vi "inferenz4.vi"(0 "fuzzified input 1":T1={"index"=-1, "fulfillment"=[], "active sets"=[3]} {"fulfillment" min=0.0 max=1.0 step=0.01 format="%.2f"}, 1 "fuzzified input 2":T1={"index"=-1, "fulfillment"=[], "active sets"=[3]} {"fulfillment" min=0.0 max=1.0 step=0.01 format="%.2f"}, 2 "fuzzified input 3":T1={"index"=-1, "fulfillment"=[], "active sets"=[3]} {"fulfillment" min=0.0 max=1.0 step=0.01 format="%.2f"}, 3 "fuzzified input 4":T1={"index"=-1, "fulfillment"=[], "active sets"=[3]} {"fulfillment" min=0.0 max=1.0 step=0.01 format="%.2f"}, 4 "Controller":T3={"Parameters"={"antecedance"=[{"ling.var."="in1", "x-min"=-1.0, "x-max"=1.0, "setarray"=[{"linguistic term"="NE1", "color"=16711680, "points"=[-1.0, -1.0, -1.0, -2.2351741790771484e-05]}, {"linguistic term"="ZE1", "color"=255, "points"=[-1.0, 0.0, 0.0, 1.0]}, {"linguistic term"="PO1", "color"=26214, "points"=[0.0, 1.0, 1.0, 1.0]}, {"linguistic term"="PB1", "color"=0, "points"=[0.009999999776482582, 0.009999999776482582, 0.009999999776482582, 0.009999999776482582]}]}, {"ling.var."="in2", "x-min"=-1.0, "x-max"=1.0, "setarray"=[{"linguistic term"="NE2", "color"=0, "points"=[0.0, 0.009999999776482582, 0.009999999776482582, 0.009999999776482582]}, {"linguistic term"="PO2", "color"=0, "points"=[0.0, 0.009999999776482582, 0.009999999776482582, 0.009999999776482582]}]}, {"ling.var."="in3", "x-min"=-1.0, "x-max"=1.0, "setarray"=[{"linguistic term"="NE1", "color"=0, "points"=[-1.0, -1.0000001192092896, -1.0000001192092896, 0.0]}, {"linguistic term"="ZE1", "color"=0, "points"=[-1.0000001192092896, 0.0, 0.0, 1.0000001192092896]}, {"linguistic term"="PO1", "color"=0, "points"=[1.4901161193847656e-08, 1.0, 1.0, 1.0000001192092896]}]}], "consequence"=[{"ling.var."="out", "x-min"=-1.0, "x-max"=1.0, "setarray"=[{"linguistic term"="NEo", "color"=16711680, "points"=[-1.0, -1.0, -1.0, 0.0]}, {"linguistic term"="ZEo", "color"=255, "points"=[-1.0, 0.0, 0.0, 1.0]}, {"linguistic term"="POo", "color"=26214, "points"=[0.0, 1.0, 1.0, 1.0]}]}], "conclusions"=[0, 1, 2, 0, 1, 2, 0, 1, 2, 2, 2, 2, 0, 0, 0, 1, 1, 1, 2, 1, 0, 2, 1, 0], "degree-of-support"=[1.0, 1.0, 1.0, 1.0, 1.0, 1.0, 1.0], "defu"=[{"inference"=0, "defumethod"=0, "modification"=TRUE, "precision"=0, "no consequence"=0, "defaultvalue"=0.0}]}, "Description"={"Info"={"Path"=path "/HD 1000/Desktop Folder/fuzzylab today/loadsave.vi", "Controller Name"="", "Date"="", "Time"=""}, "Author"="", "Text"=""}} {"Parameters"."defu"."defaultvalue" format="%.2f"; "Parameters"."degree-of-support" step=0.009999999776482582 format="%.2f"; "Parameters"."consequence"."x-min" step=0.009999999776482582 format="%.2f"; "Parameters"."consequence"."x-max" step=0.009999999776482582 format="%.2f"; "Parameters"."consequence"."setarray"."points" step=0.009999999776482582 format="%.2f"; "Parameters"."antecedance"."x-min" step=0.009999999776482582 format="%.2f"; "Parameters"."antecedance"."x-max" step=0.009999999776482582 format="%.2f"; "Parameters"."antecedance"."setarray"."points" step=0.009999999776482582 format="%.2f"}) -> (5 "fuzzified consequence":T2={"fullfilment*DoS"=[19.0, 20.0, 22.0, 23.0], "active consequence"=[19, 20, 22, 23]} {"fullfilment*DoS" format="%.2f"}, 6 "firering rules":i32[](array[numeric])=[19, 20, 22, 23], 7 "error out":errorcluster={"status"=FALSE, "code"=0, "source"="no error"})   [LabVIEW 2020, in "NI_fuzzy logic.lvlib"]
uses:
  <vilib>/addons/control/fuzzy/NI_fuzzy logic.lvlib
panel:
  in  "no error":errorcluster
  out "Minimum":dbl[](array[numeric])=[19.0, 20.0, 22.0, 23.0] format="%.2f"
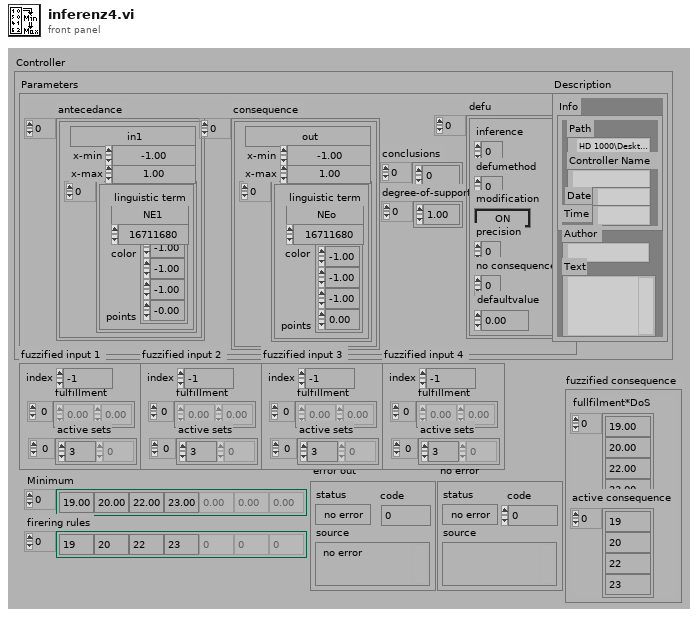
[diagram p1: front panel]
types:
  T1 = cluster{"index":i32, "fulfillment":dbl[], "active sets":i32[]}
  T2 = cluster{"fullfilment*DoS":dbl[], "active consequence":i32[]}
  T3 = cluster{"Parameters":cluster{"antecedance":cluster{"ling.var.":string, "x-min":dbl, "x-max":dbl, "setarray":cluster{"linguistic term":string, "color":u32, "points":dbl[]}[]}[], "consequence":cluster{"ling.var.":string, "x-min":dbl, "x-max":dbl, "setarray":cluster{"linguistic term":string, "color":u32, "points":dbl[]}[]}[], "conclusions":u16[], "degree-of-support":dbl[], "defu":cluster{"inference":u16, "defumethod":u16, "modification":bool, "precision":u16, "no consequence":u16, "defaultvalue":dbl}[]}, "Description":cluster{"Info":cluster{"Path":path, "Controller Name":string, "Date":string, "Time":string}, "Author":string, "Text":string}}
  T4 = cluster{"index":i32, "fulfillment":dbl[], "active sets":i32[]}[]
  T5 = cluster{"ling.var.":string, "x-min":dbl, "x-max":dbl, "setarray":cluster{"linguistic term":string, "color":u32, "points":dbl[]}[]}[]
  T6 = cluster{"ling.var.":string, "x-min":dbl, "x-max":dbl, "setarray":cluster{"linguistic term":string, "color":u32, "points":dbl[]}[]}
  T7 = cluster{"linguistic term":string, "color":u32, "points":dbl[]}[]
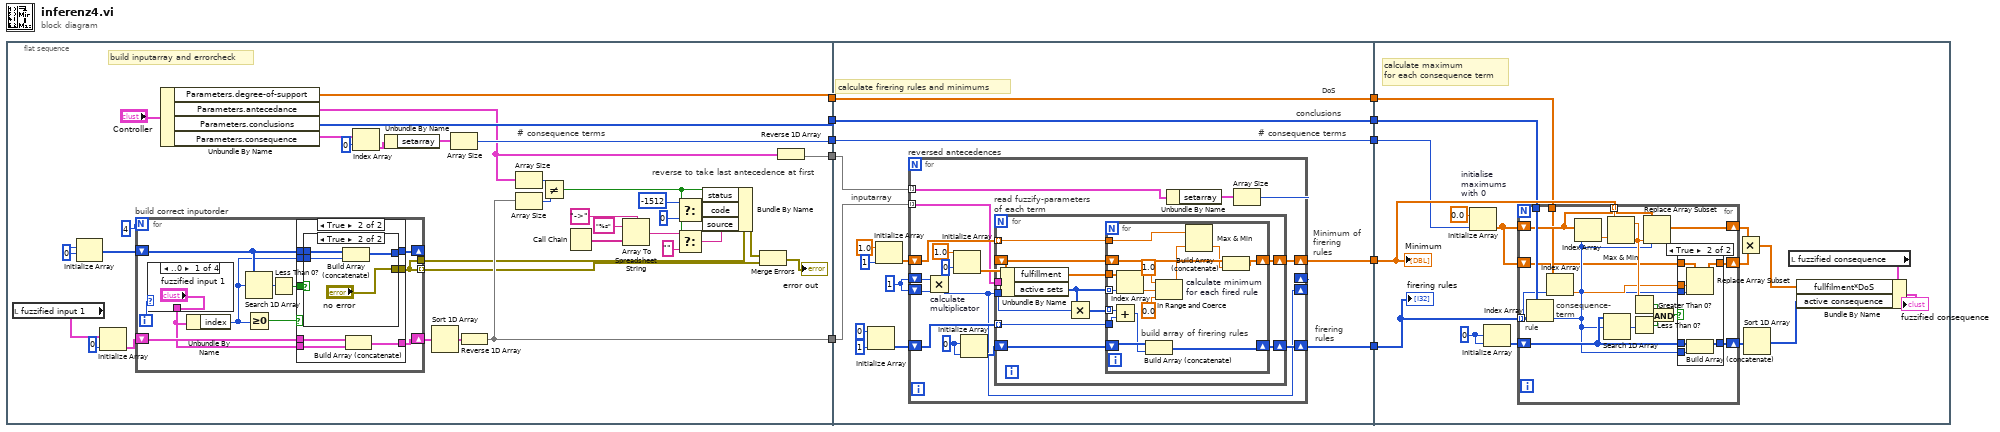
[diagram p0: block diagram]
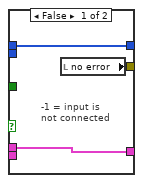
[diagram p2: hidden frame]
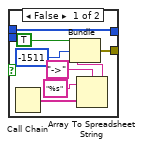
[diagram p3: hidden frame]
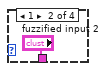
[diagram p4: hidden frame]
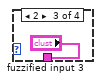
[diagram p5: hidden frame]
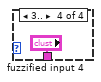
[diagram p6: hidden frame]
diagram:
  n1 = flat-sequence {
    tunnel: [w40] -> w10
    tunnel: [w41] -> w9
    tunnel: [w39] -> w8
    tunnel: [w28] -> w7
    tunnel: [w18] -> w6
    tunnel: w10 -> [w86]
    tunnel: [w86] -> w5
    tunnel: [w89] -> w4
    tunnel: [w90] -> w3
    tunnel: w9 -> [w85]
    tunnel: [w85] -> w2
    tunnel: w8 -> [w88]
    tunnel: w7 -> [w87]
    tunnel: w6 -> [w84]
    tunnel: [w84] -> w1
    tunnel: w5 -> [w151]
    tunnel: w4 -> [w152]
    tunnel: w3 -> [w149]
    tunnel: w2 -> [w150]
    tunnel: w1 -> [w143]
    frame #0 {
      w23 = 0
      # "build inputarray and errorcheck"
      # "# consequence terms"
      # "reverse to take last antecedence at first"
      n2 = local read "fuzzified input 1"() -> (w36:T1)
      n3 = Initialize Array(w23, w23) -> (w24:i32[])
      n4 = Initialize Array(w36, 0) -> (w34:T4)
      n5 = for "build correct inputorder" {
        N: 4 -> [_]
        shift-right: [w54] -> w33
        shift-left: w34 -> [w55]
        shift-right: [w49] -> _
        shift-left: w24 -> [w50]
        tunnel: [w46] -> w12 mode=indexing
        tunnel: [w46] -> w19
        i -> [w56]
        n6 = case shown="..0" w56 {
          tunnel: ["fuzzified input 1" "fuzzified input 2" "fuzzified input 3" "fuzzified input 4"] -> w53
          frame ..0 {
          }
          frame 1 {
          }
          frame 2 {
          }
          frame 3.. {
          }
        }
        n7 = Unbundle By Name(w53) -> ("index"=w48:i32)
        n8 = Search 1D Array(1D array=w50, element=w48) -> (index of element=w52:i32)  [unwired: 1 out]
        n9 = Greater Or Equal To 0?(x=w48) -> (x >= 0?=w51:bool)
        n10 = Less Than 0?(x=w52) -> (x < 0?=w47:bool)
        n11 = case shown="True" w51 {
          tunnel: w55 -> [w59 w67]
          tunnel: [w59 w66] -> w54
          tunnel: w53 -> [_ w65]
          tunnel: w50 -> [w58 w64]
          tunnel: [w58 w63] -> w49
          tunnel: w48 -> [_ w62]
          tunnel: w47 -> [_ w61]
          tunnel: [w57 w60] -> w46
          frame False {
            # "-1 = input is \nnot connected"
            n12 = local read "no error"() -> (w57:errorcluster)
          }
          frame True {
            n13 = case shown="True" w61 {
              tunnel: w64 -> [w75 w79]
              tunnel: [w75 w78] -> w63
              tunnel: w62 -> [_ w77]
              tunnel: [w72 "no error"] -> w60
              frame False {
                n14 = Call Chain() -> (call chain=w69:string[])
                n15 = Array To Spreadsheet String(delimiter (Tab)="->", array=w69, 3:"%s" ("format string")) -> (spreadsheet string=w68:string)
                n16 = Bundle(TRUE, -1511, "spreadsheet string"=w68) -> (w72:cluster{bool, i32, "spreadsheet string":string})  [unwired: 1 out]
              }
              frame True {
                n17 = Build Array (concatenate)(w79, w77) -> (w78:i32[])
              }
            }
            n18 = Build Array (concatenate)(w67, w65) -> (w66:T4)
          }
        }
      }
      n19 = Unbundle By Name("Controller") -> ("Parameters.degree-of-support"=w18:dbl[], "Parameters.antecedance"=w32:T5, "Parameters.conclusions"=w40:u16[], "Parameters.consequence"=w43:T5)
      n20 = Index Array(array=w43, index=0) -> (element=w44:T6)
      n21 = Unbundle By Name(w44) -> ("setarray"=w45:T7)
      n22 = Sort 1D Array(array=w33) -> (sorted array=w29:T4)
      n23 = Array Size(array=w45) -> (size(s)=w41:i32)
      n24 = Reverse 1D Array(array=w29) -> (reversed array=w28:T4)
      n25 = Array Size(array=w32) -> (size(s)=w31:i32)
      n26 = Array Size(array=w28) -> (size(s)=w30:i32)
      n27 = Not Equal?(x=w31, y=w30) -> (x != y?=w21:bool)
      n28 = Call Chain() -> (call chain=w15:string[])
      n29 = Array To Spreadsheet String(delimiter (Tab)="->", array=w15, 3:"%s" ("format string")) -> (spreadsheet string=w14:string)
      n30 = Select(t=-1512, s=w21, f=0) -> (s? t:f=w22:i32)
      n31 = Select(t=w14, s=w21, f="") -> (s? t:f=w20:string)
      n32 = Bundle By Name(cluster=w19, "status"=w21, "code"=w22, "source"=w20) -> (w13:errorcluster)
      n33 = Merge Errors(w13, w12) -> (→"error out":errorcluster)
      n34 = Reverse 1D Array(array=w32) -> (reversed array=w39:T5)
    }
    frame #1 {
      w94 = 1
      # "DoS"
      # "# consequence terms"
      # "conclusions"
      # "inputarray"
      # "reversed antecedences"
      # "calculate firering rules and minimums"
      # "firering\nrules"
      # "Minimum of\nfirering \nrules"
      n35 = Initialize Array(0, 1) -> (w91:i32[])
      n36 = Initialize Array(1.0, 1) -> (w97:dbl[])
      n37 = for {
        shift-right: [w113] -> w90
        shift-left: w91 -> [w112]
        shift-right: [w106] -> _
        shift-left: w94 -> [w109]
        shift-right: [w99] -> _
        shift-left: w94 -> [w108]
        tunnel: w88 -> [w105] mode=indexing
        shift-right: [w100] -> w89
        shift-left: w97 -> [w101]
        tunnel: w87 -> [w98] mode=indexing
        w111 = 0
        n38 = Multiply "calculate \nmultiplicator"(x=w109, y=w108) -> (x*y=w99:i32)
        n39 = Initialize Array(1.0, 0) -> (w102:dbl[])
        n40 = Initialize Array(w111, w111) -> (w110:i32[])
        n41 = for "read fuzzify-parameters \nof each term" {
          shift-right: [w122] -> w113
          shift-left: w110 -> [w123]
          tunnel: w112 -> [w124] mode=indexing
          tunnel: w99 -> [w121]
          tunnel: w98 -> [w120]
          shift-right: [w115] -> w100
          shift-left: w102 -> [w117]
          tunnel: w101 -> [w116] mode=indexing
          n42 = Unbundle By Name(w120) -> ("fulfillment"=w118:dbl[], "active sets"=w114:i32[])
          n43 = Multiply(x=w121, y=w114) -> (x*y=w119:i32[])
          n44 = for {
            tunnel: w124 -> [w137]
            shift-right: [w138] -> w122
            shift-left: w123 -> [w139]
            tunnel: w119 -> [w131] mode=indexing
            tunnel: w118 -> [w135]
            tunnel: w116 -> [w134]
            shift-right: [w132] -> w115
            shift-left: w117 -> [w133]
            tunnel: w114 -> [w130] mode=indexing
            # "build array of firering rules"
            n45 = Add(x=w131, y=w137) -> (x+y=w136:i32)
            n46 = Index Array(array=w135, index=w130) -> (element=w128:dbl)
            n47 = Build Array (concatenate)(w139, w136) -> (w138:i32[])
            n48 = In Range and Coerce(upper limit=1.0, x=w128, lower limit=0.0 ("upper limit")) -> (coerced(x)=w125:dbl)  [unwired: 1 out]
            n49 = Max & Min "calculate minimum \nfor each fired rule"(x=w134, y=w125) -> (min(x,y)=w129:dbl)  [unwired: 1 out]
            n50 = Build Array (concatenate)(w133, w129) -> (w132:dbl[])
          }
        }
        n51 = Unbundle By Name(w105) -> ("setarray"=w107:T7)
        n52 = Array Size(array=w107) -> (size(s)=w106:i32)
      }
    }
    frame #2 {
      w154 = 0
      # "calculate maximum \nfor each consequence term"
      n53 = Initialize Array "initialise \nmaximums \nwith 0"(0.0, w150) -> (w144:dbl[])
      n54 = Initialize Array(w154, w154) -> (w155:i32[])
      n55 = for "calculate maximum \nfor each consequenceterm" {
        tunnel: w149 -> [w161] mode=indexing
        tunnel: w151 -> [w173]
        shift-right: [w169] -> w142
        shift-left: w144 -> [w170]
        tunnel: w152 -> [w171] mode=indexing
        shift-right: [w167] -> w146
        shift-left: w155 -> [w163]
        shift-right: [w156] -> w141
        shift-left: w144 -> [w157]
        tunnel: w143 -> [w160]
        # "consequence-\nterm"
        # "rule"
        n56 = Index Array(array=w173, index=w161) -> (element=w158:u16)
        n57 = Index Array(array=w160, index=w161) -> (element=w159:dbl)
        n58 = Index Array(array=w170, index=w158) -> (element=w172:dbl)
        n59 = Search 1D Array(1D array=w163, element=w158) -> (index of element=w166:i32)  [unwired: 1 out]
        n60 = Max & Min(x=w171, y=w172) -> (max(x,y)=w168:dbl)  [unwired: 1 out]
        n61 = Greater Than 0?(x=w168) -> (x > 0?=w165:bool)
        n62 = Less Than 0?(x=w166) -> (x < 0?=w162:bool)
        n63 = Replace Array Subset(array=w170, new element=w168, index=w158) -> (w169:dbl[])
        n64 = And(x=w165, y=w162) -> (x .and. y?=w164:bool)
        n65 = case shown="True" w164 {
          tunnel: [w175 w182] -> w167
          tunnel: w163 -> [w175 w181]
          tunnel: w158 -> [_ w180]
          tunnel: w159 -> [_ w179]
          tunnel: w158 -> [_ w178]
          tunnel: w157 -> [w174 w177]
          tunnel: [w174 w176] -> w156
          frame False {
          }
          frame True {
            n66 = Replace Array Subset(array=w177, new element=w179, index=w178) -> (w176:dbl[])
            n67 = Build Array (concatenate)(w181, w180) -> (w182:i32[])
          }
        }
      }
      n68 = Multiply(x=w142, y=w141) -> (x*y=w140:dbl[])
      n69 = Sort 1D Array(array=w146) -> (sorted array=w145:i32[])
      n70 = local read "fuzzified consequence"() -> (w148:T2)
      n71 = Bundle By Name(cluster=w148, "fullfilment*DoS"=w140, "active consequence"=w145) -> (→"fuzzified consequence":T2)
      "firering rules" <- w149
      "Minimum" <- w152
    }
  }
